vi "AngleBetween2Vectors.vi"(8 "error in (no error)":errorcluster, 9 "Array 1":dbl[](array[numeric]), 10 "Array 2":dbl[](array[numeric]), 11 "Utilities in":refnum<class "Utilities.lvclass">) -> (0 "error out":errorcluster, 2 "Numeric":dbl, 3 "Utilities out":refnum<class "Utilities.lvclass">)   [LabVIEW 2023, in "Utilities.lvclass"]
uses:
  Utilities.lvclass
  <vilib>/Analysis/baseanly.llb/Real Dot Product.vi
  <vilib>/Analysis/NI_AALBase.lvlib
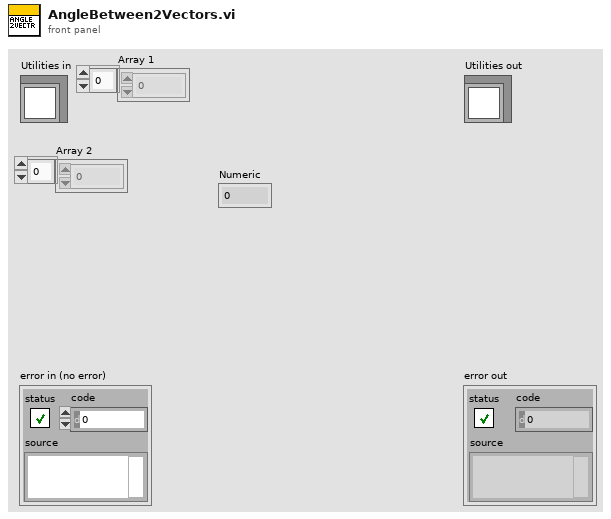
[diagram p1: front panel]
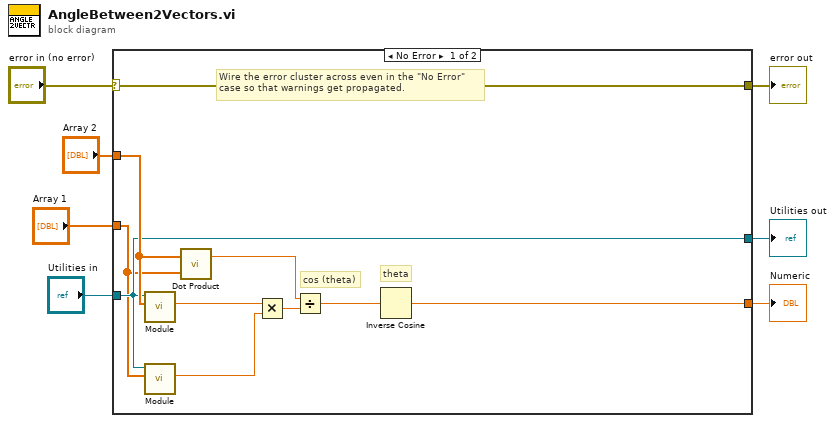
[diagram p0: block diagram]
diagram:
  n1 = case shown="No Error" "error in (no error)" {
    selector: "error in (no error)" -> [w17 w19]
    tunnel: [w17 w19] -> w6
    tunnel: [w9 w18] -> w4
    tunnel: "Utilities in" -> [w9 w18]
    tunnel: [w11 _] -> w3
    tunnel: "Array 2" -> [w10 _]
    tunnel: "Array 1" -> [w8 _]
    frame No Error {
      # "theta"
      # "cos (theta)"
      # "Wire the error cluster across even in the \"No Error\"\ncase so that warnings get propagated."
      n2 = call-dynamic "Module.vi"("2D vector"=w10, "Utilities in"=w9) -> ("Modulo"=w13:dbl)  [unwired: 7 in, 2 out]
      n3 = call-dynamic "Module.vi"("2D vector"=w8, "Utilities in"=w9) -> ("Modulo"=w12:dbl)  [unwired: 7 in, 2 out]
      n4 = call-poly <vilib>:"Dot Product.vi"("Y Vector"=w8, "X Vector"=w10) -> ("X * Y"=w14:dbl)  [unwired: 1 out]
      n5 = Multiply(x=w13, y=w12) -> (x*y=w15:dbl)
      n6 = Divide(x=w14, y=w15) -> (x/y=w16:dbl)
      n7 = Inverse Cosine(1:w16) -> (0:w11:dbl)
    }
    frame Error {
    }
  }
  "error out" <- w6
  "Utilities out" <- w4
  "Numeric" <- w3
